vi "ECU Selector.vi"(6 "Model":string) -> (0 "ID Response":string, 1 "Puerto DAQ":i32, 2 "Numeric Request":i32=416962034 format="%x", 3 "ID Request":string, 4 "frame":refnum<k21>="Escritura_Driver\nElatch Database")   [LabVIEW 2023]
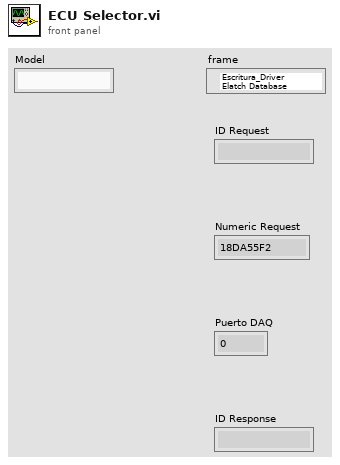
[diagram p1: front panel]
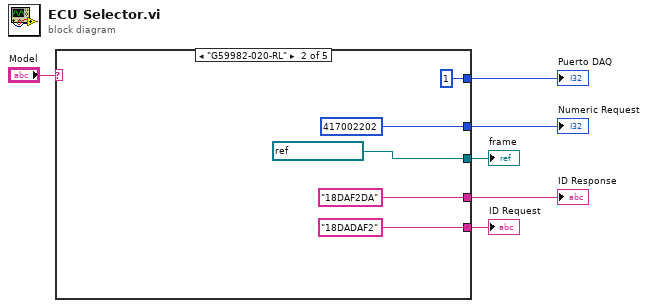
[diagram p0: block diagram]
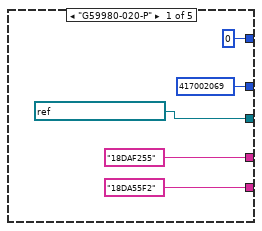
[diagram p2: hidden frame]
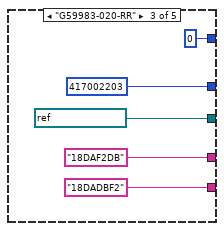
[diagram p3: hidden frame]
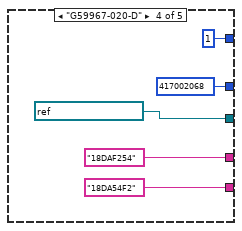
[diagram p4: hidden frame]
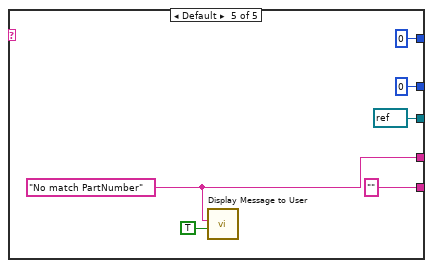
[diagram p5: hidden frame]
diagram:
  n1 = case shown="\"G59982-020-RL\"" "Model" {
    tunnel: ["18DA55F2" "18DADAF2" "18DADBF2" "18DA54F2" ""] -> w6
    tunnel: ["18DAF255" "18DAF2DA" "18DAF2DB" "18DAF254" w27] -> w5
    tunnel: [417002069 417002202 417002203 417002068 0] -> w4
    tunnel: [refnum<k21> "Escritura_Passenger\nElatch Database" ("frame") refnum<k21> "Escritura_RL\nElatch Database" ("frame") refnum<k21> "Escritura_RR\nElatch Database" ("frame") refnum<k21> "Escritura_Driver\nElatch Database" ("frame") refnum<k21> refnum ("frame")] -> w3
    tunnel: [0 1 0 1 0] -> w2
    frame "G59980-020-P" {
    }
    frame "G59982-020-RL" {
    }
    frame "G59983-020-RR" {
    }
    frame "G59967-020-D" {
    }
    frame Default {
      w27 = "No match PartNumber" ("Message")
      n2 = call "Display Message to User"("Enable"=TRUE, "Message"=w27) -> ()  [unwired: 8 in, 2 out]
    }
  }
  "ID Request" <- w6
  "ID Response" <- w5
  "Numeric Request" <- w4
  "frame" <- w3
  "Puerto DAQ" <- w2
